vi "filter data.vi"(6 "Filter? (F)":bool, 9 "History":sgl[](array[numeric])=[0.0, 0.0, 0.0, 0.0], 11 "New readings":sgl[](array[numeric])=[0.0, 0.0, 0.0, 0.0]) -> (3 "output":sgl[](array[numeric]))   [LabVIEW 2018]
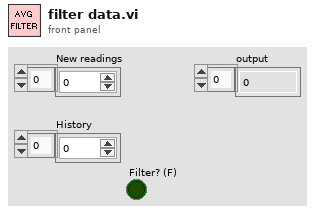
[diagram p1: front panel]
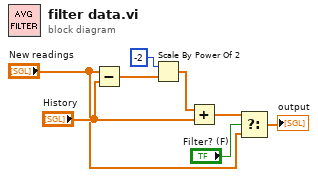
[diagram p0: block diagram]
diagram:
  n1 = Subtract(x="New readings", y="History") -> (x-y=w5:sgl[])
  n2 = Scale By Power Of 2(n=i16 -2, x=w5) -> (x*2^n=w7:sgl[])
  n3 = Add(x=w7, y="History") -> (x+y=w4:sgl[])
  n4 = Select(t=w4, s="Filter? (F)", f="New readings") -> (s? t:f=→"output":sgl[])
